vi "XIPIN_Triple-Rate_SDI_1_0.vi"   [LabVIEW 2017]
doc: "Triple-Rate SDI RX/TX Interface supporting SD-SDI, HD-SDI, and 3G-SDI for Virtex-6 GTX transceivers.\n------------------------------------\n<b>Need License</b> : No"
uses:
  <vilib>/rvi/XilinxIP/XIPIN_XNode/niFpgaXIPIN.xnode
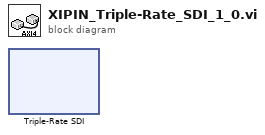
[diagram p0: block diagram]
diagram:
  n1 = xnode ("Triple-Rate SDI")() -> ()
